vi "libssh2_knownhost_writefile.vi"(8 "error in (no error)":errorcluster, 9 "type (OpenSSH)":T1, 10 "filename":path, 11 "host key database":T2) -> (0 "error out":errorcluster)   [LabVIEW 2013, in "libssh2.lvlib"]
doc: "Write a host key database to a file."
uses:
  libssh2.lvlib
  Host Key Database Refnum.ctl
  Host Key File Type.ctl
  Not A Host Key Database.vi
  <vilib>/Utility/error.llb/Error Cluster From Error Code.vi
  Global Settings.vi
  Read Host Key Database Refnum.vi
  <vilib>/Utility/semaphor.llb/Acquire Semaphore.vi
  <vilib>/Utility/semaphor.llb/Release Semaphore.vi
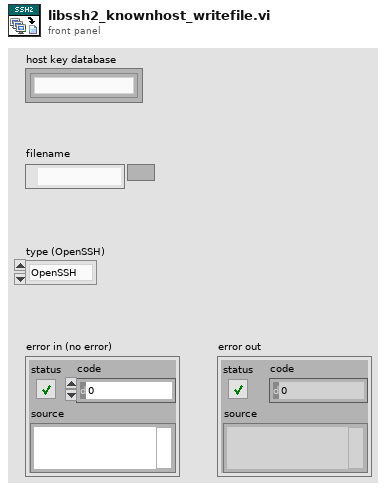
[diagram p1: front panel]
types:
  T1 = typedef "libssh2.lvlib/Host Key File Type.ctl" = enum16{"OpenSSH"}
  T2 = typedef "libssh2.lvlib/Host Key Database Refnum.ctl" = refnum<k1>
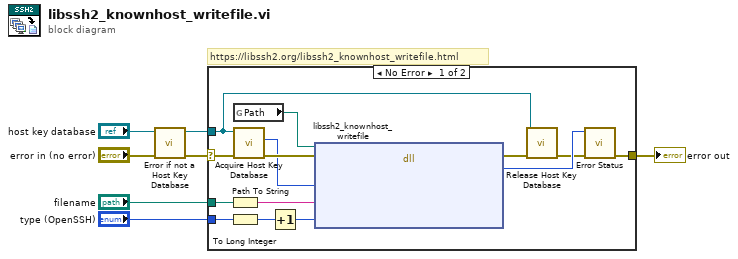
[diagram p0: block diagram]
diagram:
  # "https://libssh2.org/libssh2_knownhost_writefile.html"
  n1 = call "Error if not a Host Key Database.vi"("error in (no error)"="error in (no error)", "host key database"="host key database") -> ("error out"=w3:errorcluster, "host key database out"=w1:T2)  [unwired: 8 in]
  n2 = case shown="No Error" w3 {
    selector: w3 -> [w19 w22]
    tunnel: [w18 w22] -> w7
    tunnel: "filename" -> [w21 _]
    tunnel: "type (OpenSSH)" -> [w20 _]
    tunnel: w1 -> [w8 _]
    frame No Error {
      n3 = Path To String(path=w21) -> (string=w12:string)
      n4 = To Long Integer(number=w20) -> (32bit integer=w11:i32)
      n5 = global read "Global Settings.vi" "Path"() -> (w14:path)
      n6 = call "Acquire Host Key Database.vi"("error in (no error)"=w19, "host key database"=w8) -> ("error out"=w16:errorcluster, "LIBSSH2_KNOWNHOSTS*"=w15:u64)  [unwired: 8 in]
      n7 = Increment(x=w11) -> (x+1=w10:i32)
      n8 = dll-call lib="?" fn="libssh2_knownhost_writefile"(path in=w14, error in=w16, "hosts"=w15, "filename"=w12, "type"=w10) -> (error out=w17:errorcluster, "return value"=w13:i32)  [unwired: 4 in, 1 out]
      n9 = call "Release Host Key Database.vi"("error in (no error)"=w17, "host key database"=w8) -> ("error out"=w9:errorcluster)  [unwired: 9 in]
      n10 = call "Error Status.vi"("error in (no error)"=w9, "return value"=w13) -> ("error out"=w18:errorcluster)  [unwired: 8 in, 1 out]
    }
    frame Error {
    }
  }
  "error out" <- w7
